vi "libcheck_descriptor.vi"(8 "error in (no error)":errorcluster, 10 "Descriptor":string) -> (0 "error out":errorcluster, 2 "result":string)   [LabVIEW 2015]
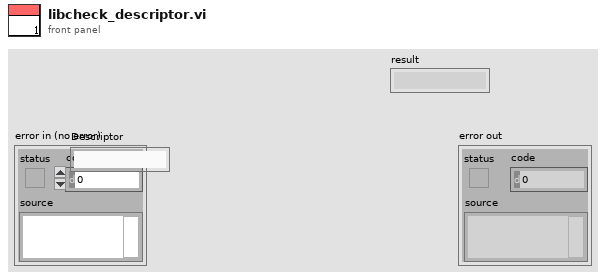
[diagram p1: front panel]
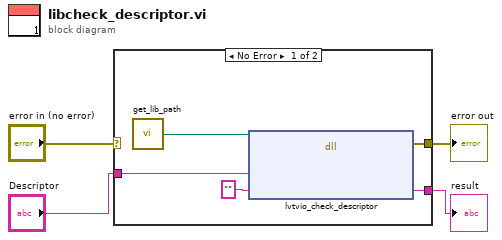
[diagram p0: block diagram]
diagram:
  n1 = case shown="No Error" "error in (no error)" {
    selector: "error in (no error)" -> [_ w10]
    tunnel: [w8 w10] -> w1
    tunnel: "Descriptor" -> [w7 _]
    tunnel: [w5 _] -> w3
    frame No Error {
      n2 = call "get_lib_path.vi"() -> ("Path"=w9:path)
      n3 = dll-call lib="S:/thingiverselv/lib/liblvtvio.dll" fn="lvtvio_check_descriptor"(path in=w9, "descriptor"=w7, "result"="") -> (error out=w8:errorcluster, "result"=w5:string)  [unwired: 4 in, 1 out]
    }
    frame Error {
    }
  }
  "error out" <- w1
  "result" <- w3
